vi "is_sweep_finished.vi"(8 "error in (no error)":errorcluster, 11 "ExperimentControllerDL090130Interval in":refnum<class "ExperimentControllerDL090130Interval.lvclass">) -> (0 "error out":errorcluster, 2 "sweep finished?":bool, 3 "ExperimentControllerDL090130Interval out":refnum<class "ExperimentControllerDL090130Interval.lvclass">)   [LabVIEW 2010]
uses:
  ExperimentControllerDL090130Interval.lvclass
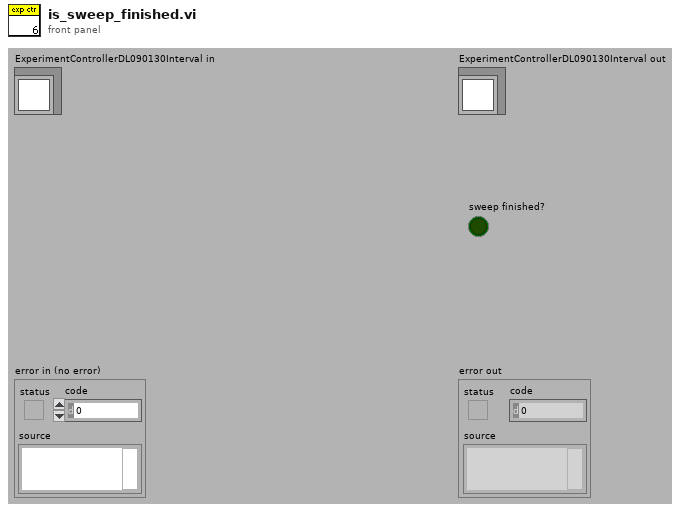
[diagram p1: front panel]
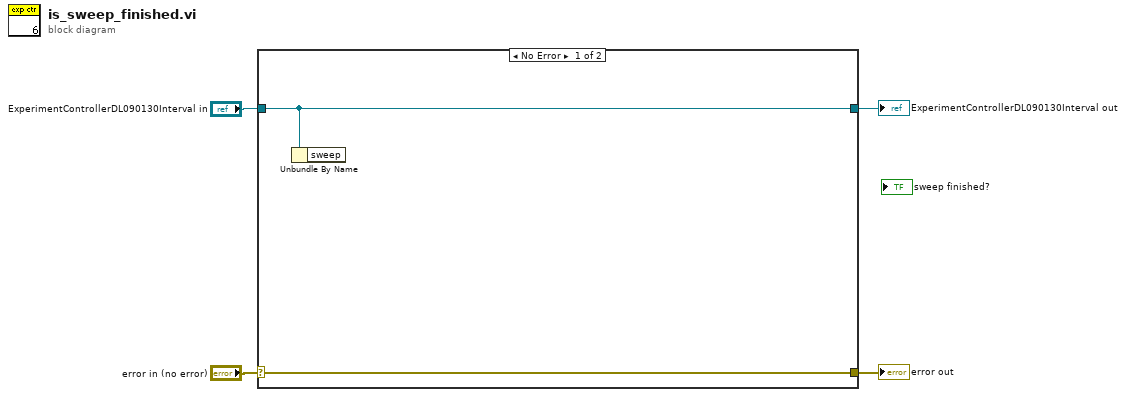
[diagram p0: block diagram]
diagram:
  n1 = case shown="No Error" "error in (no error)" {
    selector: "error in (no error)" -> [w6 w8]
    tunnel: [w6 w8] -> w3
    tunnel: [w5 w7] -> w1
    tunnel: "ExperimentControllerDL090130Interval in" -> [w5 w7]
    frame No Error {
      n2 = Unbundle By Name(w5) -> ()  [unwired: 1 out]
    }
    frame Error {
    }
  }
  "error out" <- w3
  "ExperimentControllerDL090130Interval out" <- w1
